vi "Get Protocol Type.vi"(8 "error in (no error)":errorcluster, 11 "AK RS-xxx in":refnum<class "AK RS-xxx.lvclass">) -> (0 "error out":errorcluster, 2 "protocol type":T1=enum."AK RS-XXX", 3 "AK RS-xxx out":refnum<class "AK RS-xxx.lvclass">)   [LabVIEW 2023, in "Protocols.lvlib" / "AK RS-xxx.lvclass"]
doc: "Returns AK-RS-XXX protocol type Enum."
uses:
  AK RS-xxx.lvclass
  Protocol Parent/Types/Protocol Type.ctl
  Protocol Parent/Protocol Parent.lvclass
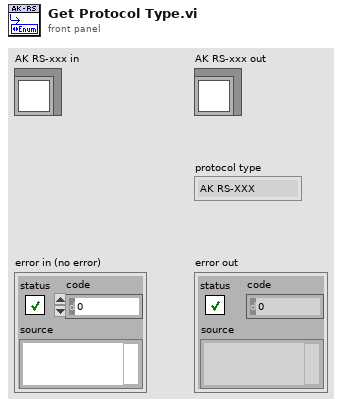
[diagram p1: front panel]
types:
  T1 = typedef "Protocols.lvlib/Protocol Parent.lvclass/Protocol Type.ctl" = enum16{"RS-XXX", "AK RS-XXX", "VISA", "TCPIP", "AK TCPIP", "UDP", "GPIB ConvBox"}
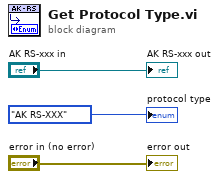
[diagram p0: block diagram]
diagram:
  "error out" <- "error in (no error)"
  "AK RS-xxx out" <- "AK RS-xxx in"
  "protocol type" <- Protocol_Type."AK RS-XXX" ("Protocol out")
